vi "LeCroy 8404MR VISA Test.vi"() -> ()   [LabVIEW 2018]
uses:
  <instrlib>/LeCroy Wave Series/Public/Data/Read Single Waveform.vi
  <instrlib>/LeCroy Wave Series/LeCroy Wave Series.lvlib
panel:
  out "Waveform Data":waveform(dbl)(graph)
  out "error out":errorcluster
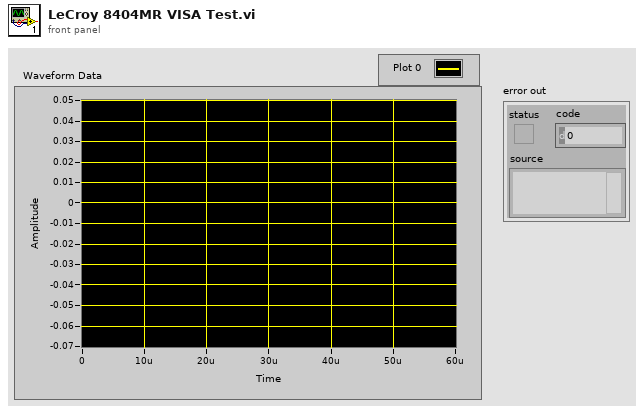
[diagram p1: front panel]
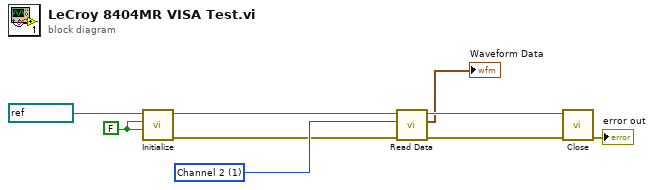
[diagram p0: block diagram]
diagram:
  w3 = u16 1 items=["Channel 1", "Channel 2", "Channel 3", "Channel 4", "Memory 1", "Memory 2", "Memory 3", "Memory 4", "Function 1", "Function 2", "Function 3", "Function 4", "Function 5", "Function 6", "Function 7", "Function 8", "Other"] ("Source (0: Channel 1)")
  w7 = FALSE ("Reset? (T: Yes)")
  n1 = call <instrlib>:"Initialize.vi"("Reset? (T: Yes)"=w7, "ID Query? (T: Yes)"=w7, "VISA resource name"=refnum<visa-resource-name> "LeCroy") -> ("error out"=w1:errorcluster, "VISA resource name out"=w2:refnum<visa-resource-name>)  [unwired: 7 in]
  n2 = call-poly <instrlib>:"Read Data.vi"("error in (no error)"=w1, "Source (0: Channel 1)"=w3, "VISA resource name"=w2) -> ("error out"=w5:errorcluster, "Waveform Data"=→"Waveform Data":waveform(dbl), "VISA resource name out"=w6:refnum<visa-resource-name>)  [unwired: 6 in]
  n3 = call <instrlib>:"Close.vi"("error in (no error)"=w5, "VISA resource name"=w6) -> ("error out"=→"error out":errorcluster)  [unwired: 9 in]
